vi "Pathfinder.vi"() -> ()   [LabVIEW 2020, in "Data.PG.lvclass"]
uses:
  Data.PG.lvclass
panel:
  out "path_to_selected_column":string="llab_038:d001(TEST_TABLE--new_stuff(hippos))"
  out "table selected":string="TEST_TABLE"
  in  "columns_list":i32(listbox)=1
  in  "Get path":bool
  in  "tables_list":i32(listbox)=34
  in  "STOP":bool
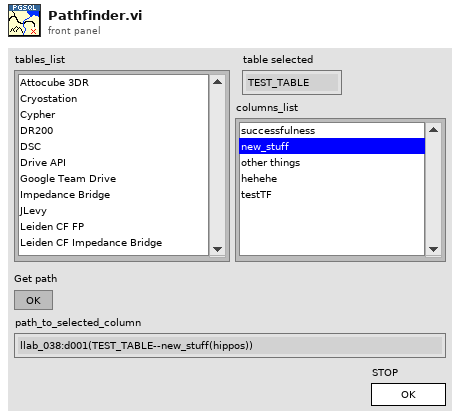
[diagram p1: front panel]
types:
  T1 = enum32{"Invalid", "Standard", "Closed", "Hidden", "Minimized", "Maximized"}
  T2 = enum32{"invalid app kind", "Development System", "Run Time System", "Student Edition", "Embedded LabVIEW", "Evaluation", "Custom"}
  T3 = cluster{"Core":cluster{"Current VI Reference":refnum<vi>, "Close Panel on Exit?":bool}, "Data.PG in":refnum<class "Data.PG.lvclass">, "connection info":cluster{"host":string, "port":string, "dbname":string, "user":string, "password":string}, "table names":string[], "table paths":string[], "column names":string[], "column units":string[], "column paths":string[], "new table name":string, "new column name":string, "new column data type":string, "new column units":string, "selected table":string, "selected column":string, "selected table path":string, "selected column path":string, "Start":timestamp, "End":timestamp, "max points":i32, "selected column units":string}
  T4 = cluster{"host":string, "port":string, "dbname":string, "user":string, "password":string}
  T5 = cluster{"Current VI Reference":refnum<vi>, "Close Panel on Exit?":bool}
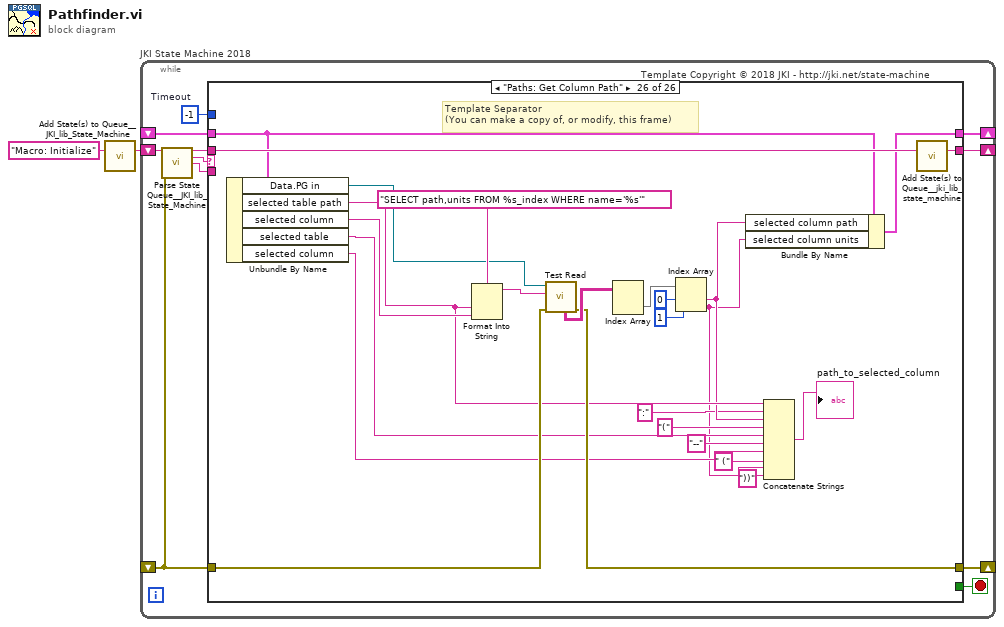
[diagram p0: block diagram]
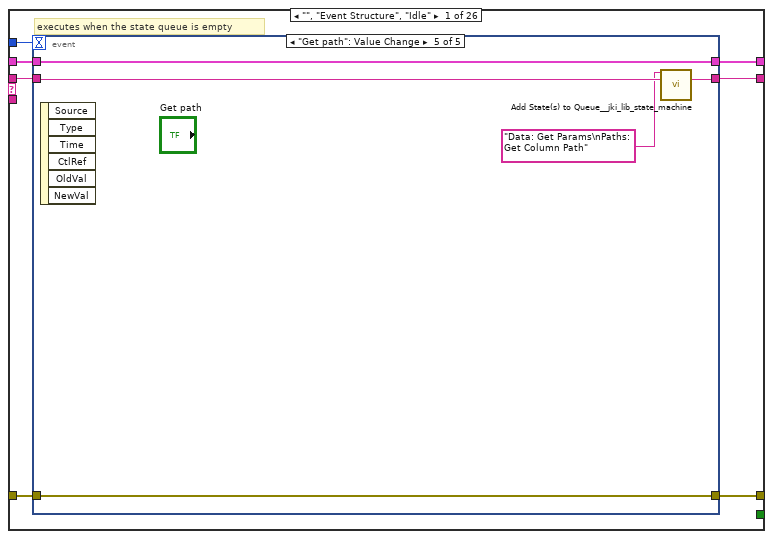
[diagram p2: hidden frame]
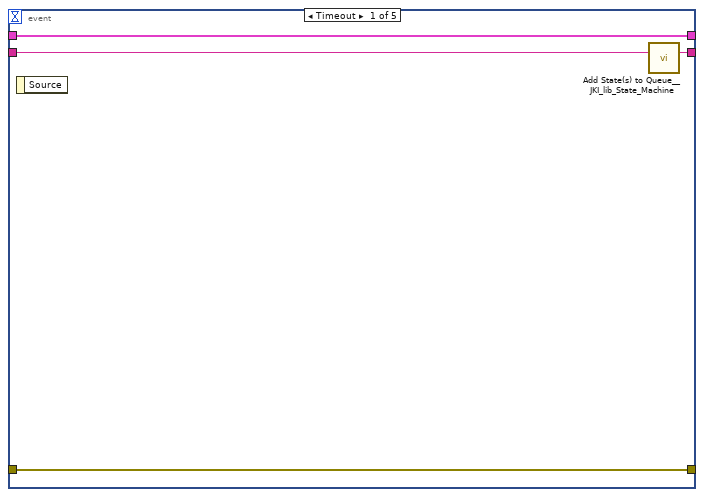
[diagram p3: hidden frame]
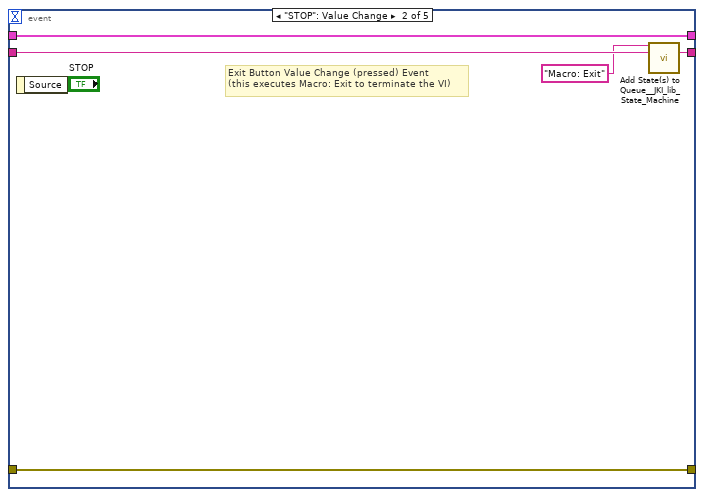
[diagram p4: hidden frame]
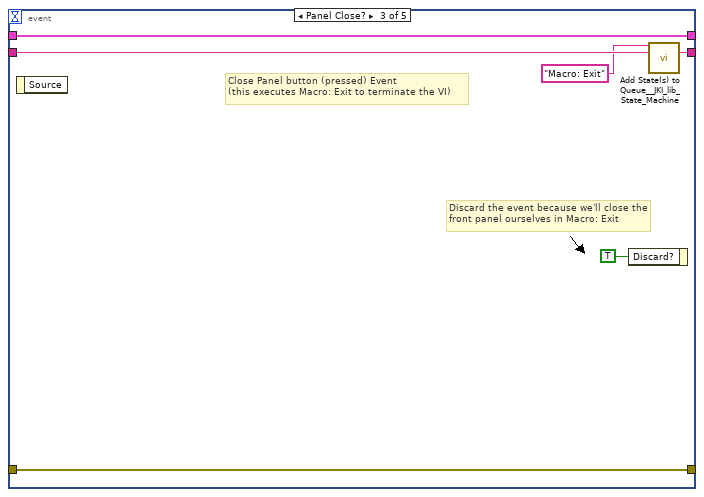
[diagram p5: hidden frame]
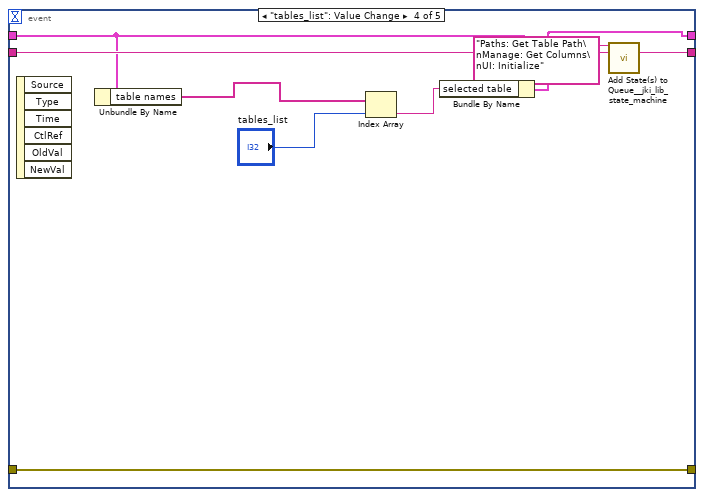
[diagram p6: hidden frame]
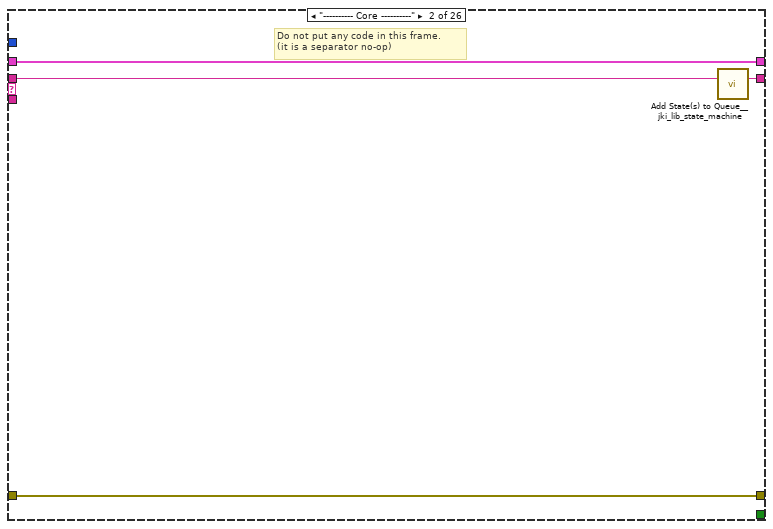
[diagram p7: hidden frame]
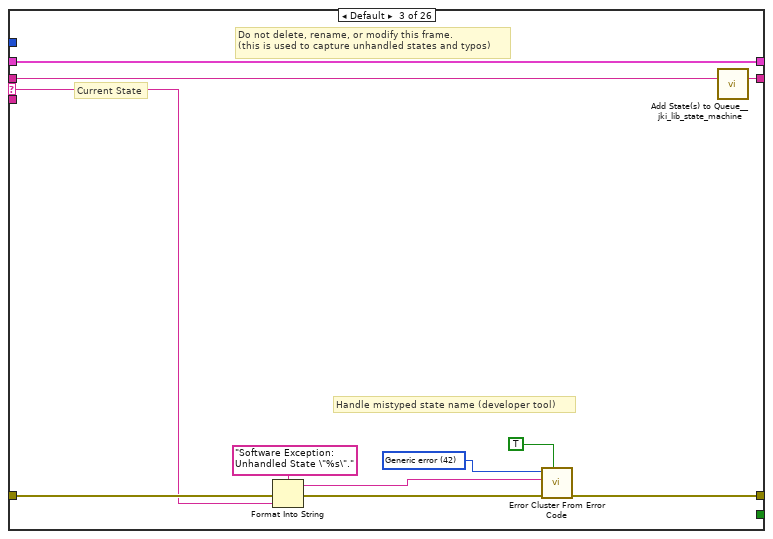
[diagram p8: hidden frame]
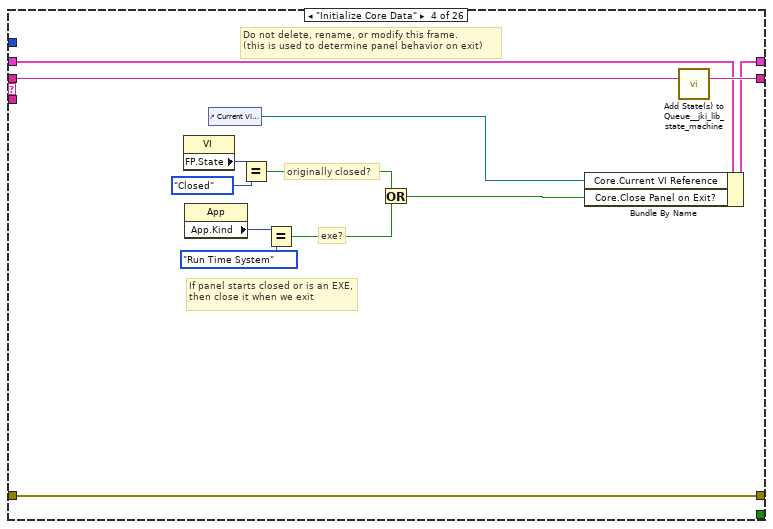
[diagram p9: hidden frame]
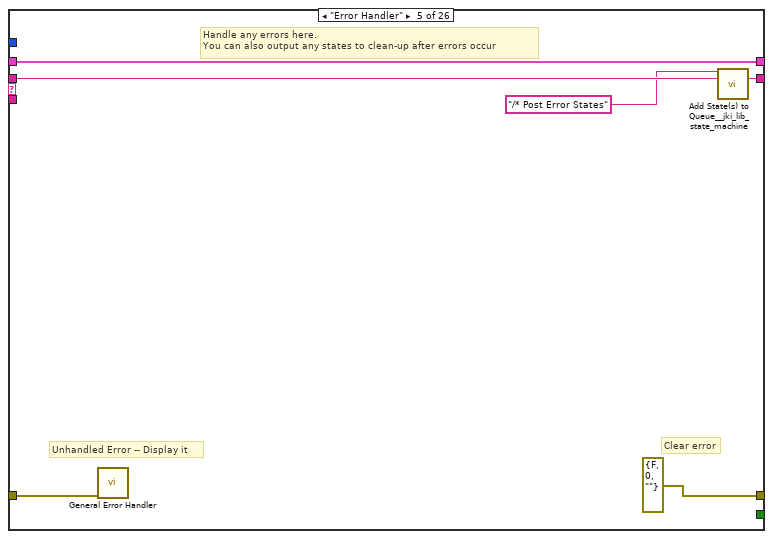
[diagram p10: hidden frame]
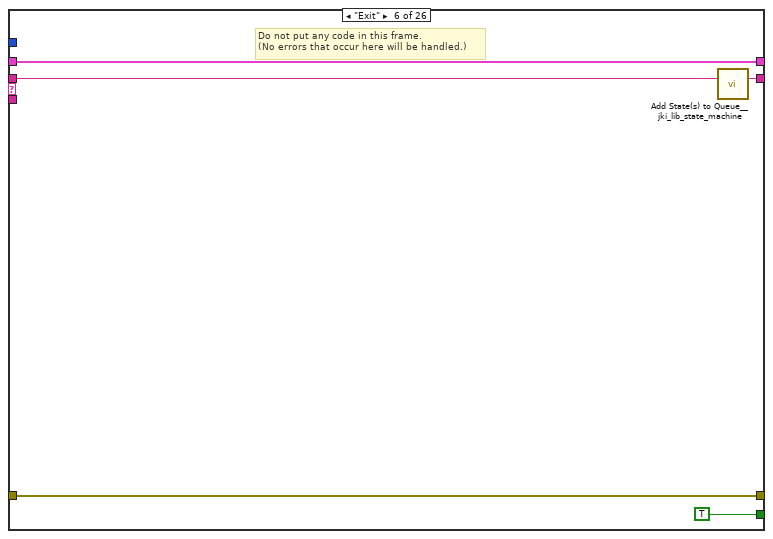
[diagram p11: hidden frame]
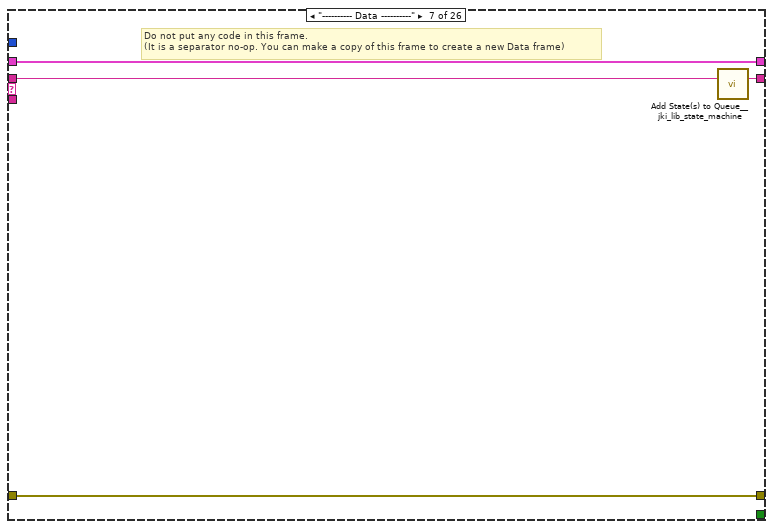
[diagram p12: hidden frame]
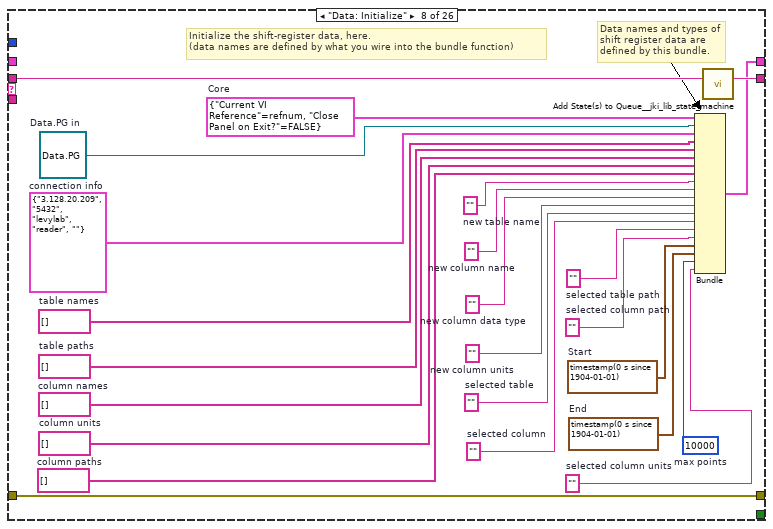
[diagram p13: hidden frame]
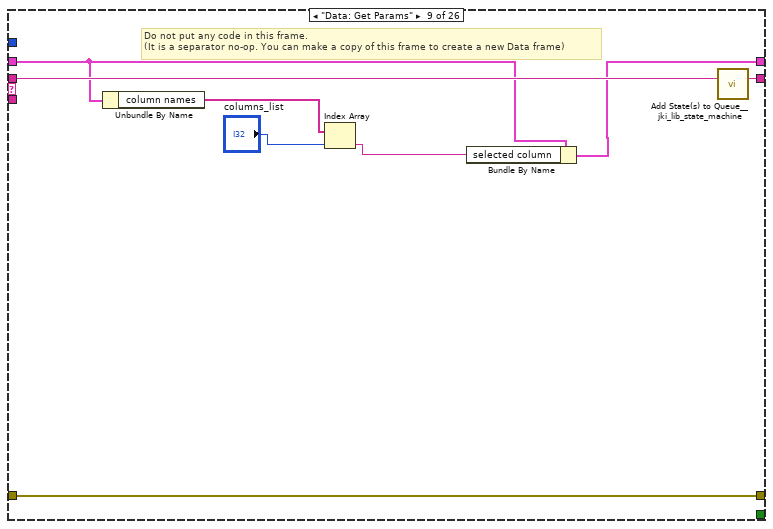
[diagram p14: hidden frame]
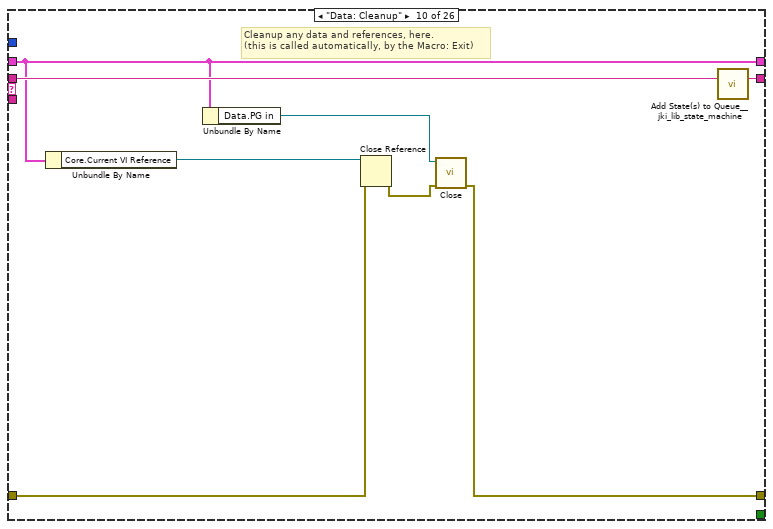
[diagram p15: hidden frame]
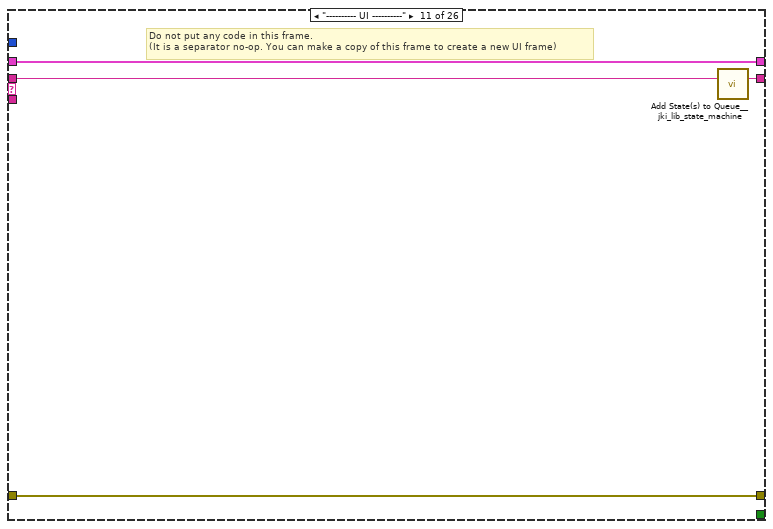
[diagram p16: hidden frame]
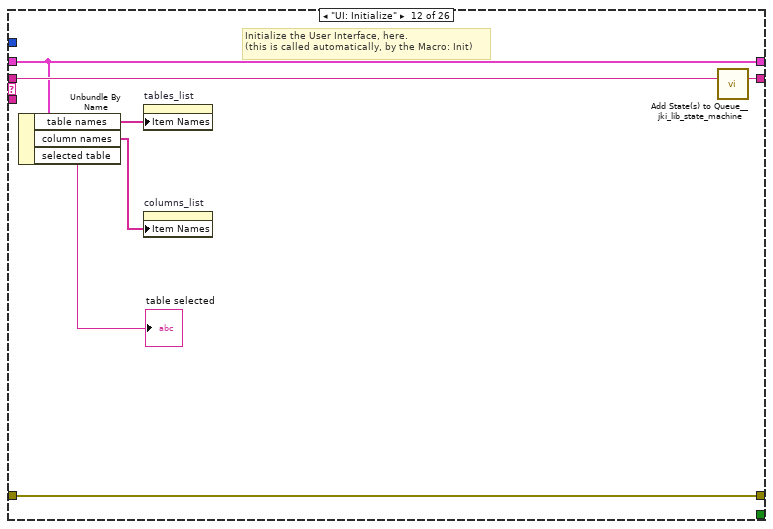
[diagram p17: hidden frame]
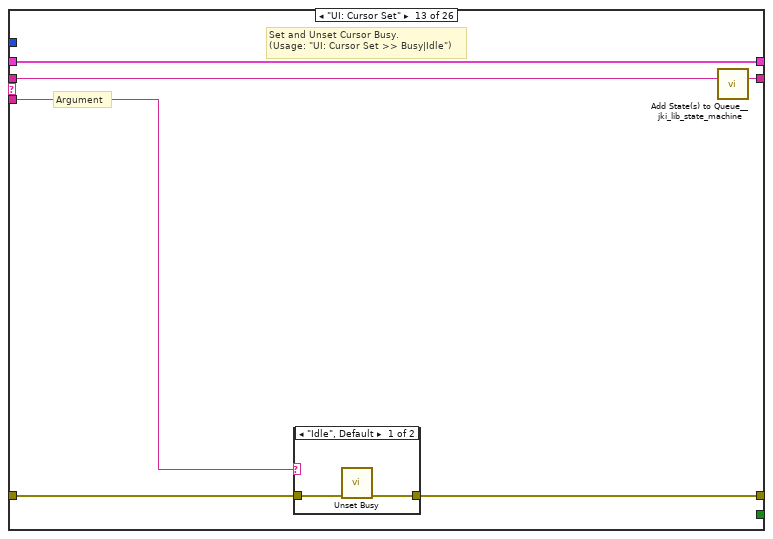
[diagram p18: hidden frame]
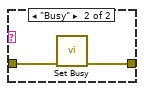
[diagram p19: hidden frame]
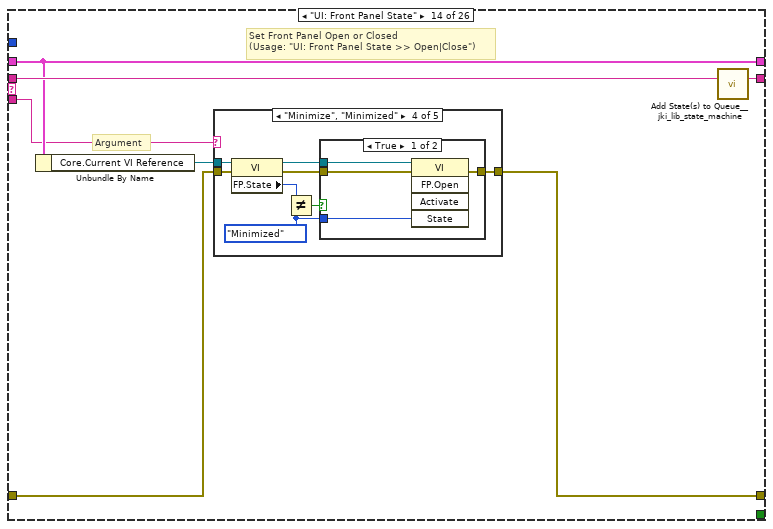
[diagram p20: hidden frame]
diagram:
  n1 = call <vilib>:"Add State(s) to Queue__JKI_lib_State_Machine.vi"("State(s) in (\"\")"="Macro: Initialize") -> ("States Out"=w2:string)  [unwired: 14 in]
  n2 = while "JKI State Machine 2018" {
    shift-right: [w6] -> _
    shift-left: _ -> [w5]
    shift-right: [w9] -> _
    shift-left: _ -> [w3]
    shift-right: [w8] -> _
    shift-left: w2 -> [w10]
    stop <- w7 stop-if-true
    w4 = -1  # Timeout
    # "Template Copyright © 2018 JKI - http://jki.net/state-machine"
    n3 = call <vilib>:"Parse State Queue__JKI_lib_State_Machine.vi"("State Queue"=w10, "Error In (no error)"=w3) -> ("Remaining States"=w12:string, "Current State"=w13:string, "Arguments"=w11:string)  [unwired: 11 in]
    n4 = case shown="\"Paths: Get Column Path\"" w13 {
      selector: w13 -> [_ _ w54 _ _ _ _ _ _ _ _ _ _ _ _ _ _ _ _ _ _ _ _ _ _ _]
      tunnel: w12 -> [w20 w53 w58 w77 w83 w88 w92 w116 w124 w132 w136 w143 w149 w160 w229 w234 w244 w248 w261 w280 w284 w290 w299 w303 w316 w341]
      tunnel: w11 -> [_ _ _ _ _ _ _ _ _ _ _ _ w144 w154 _ _ _ _ _ _ _ _ _ _ _ _]
      tunnel: w5 -> [w18 w50 w56 w70 w80 w86 w89 _ w120 w126 w133 w138 w147 w156 w226 w231 w241 w245 w253 w269 w281 w288 w293 w300 w308 w334]
      tunnel: [w17 w51 w60 w74 errorcluster {"status"=FALSE, "code"=0, "source"=""} ("error out") w85 w90 w113 w122 w127 w134 w141 w145 w157 w227 w232 w242 w246 w255 w263 w282 w285 w294 w301 w304 w331] -> w9
      tunnel: w3 -> [w16 w51 w59 w74 w79 w85 w90 w113 w122 w129 w134 w141 w146 w158 w227 w232 w242 w246 w256 w264 w282 w286 w295 w301 w305 w332]
      tunnel: [w19 w52 w57 w76 w82 w87 w91 w115 w123 w131 w135 w142 w148 w159 w228 w233 w243 w247 w260 w279 w283 w289 w298 w302 w315 w340] -> w8
      tunnel: [_ _ _ _ _ TRUE _ _ _ _ _ _ _ _ _ _ _ _ _ _ _ _ _ _ _ _] -> w7
      tunnel: [w15 w50 w56 w75 w80 w86 w89 w114 w121 w126 w133 w138 w147 w156 w226 w231 w241 w245 w252 w268 w281 w288 w292 w300 w307 w333] -> w6
      tunnel: w4 -> [w14 _ _ _ _ _ _ _ _ _ _ _ _ _ _ _ _ _ _ _ _ _ _ _ _ _]
      frame "", "Event Structure", "Idle" {
        # "executes when the state queue is empty"
        n5 = event shown="[4] \"Get path\": Value Change" {
          selector: _ -> [_ _ _ _ _]
          dyn-events: _ -> [_ _ _ _ _]
          timeout: w14 -> [_ _ _ _ _]
          tunnel: w20 -> [w24 w29 w35 w42 w47]
          tunnel: [w23 w28 w34 w43 w48] -> w19
          tunnel: w18 -> [w21 w26 w32 w38 w49]
          tunnel: [w22 w27 w33 w44 w45] -> w17
          tunnel: w16 -> [w22 w27 w33 w44 w45]
          tunnel: [w21 w26 w32 w37 w49] -> w15
          event Timeout {
            n6 = event-data() -> ()  [unwired: 1 in, 1 out]
            n7 = call <vilib>:"Add State(s) to Queue__JKI_lib_State_Machine.vi"("State(s) in (\"\")"=w24) -> ("States Out"=w23:string)  [unwired: 14 in]
          }
          event "STOP": Value Change {
            # "Exit Button Value Change (pressed) Event\n(this executes Macro: Exit to terminate the VI)"
            n8 = event-data() -> ()  [unwired: 1 in, 1 out]
            n9 = call <vilib>:"Add State(s) to Queue__JKI_lib_State_Machine.vi"("State(s) in Front (\"\")"="Macro: Exit", "State(s) in (\"\")"=w29) -> ("States Out"=w28:string)  [unwired: 13 in]
          }
          event Panel Close? {
            # "Discard the event because we'll close the front panel ourselves in Macro: Exit"
            # "Close Panel button (pressed) Event\n(this executes Macro: Exit to terminate the VI)"
            n10 = event-data() -> ()  [unwired: 1 in, 1 out]
            n11 = event-data("Discard?"=TRUE) -> ()  [unwired: 1 in, 1 out]
            n12 = call <vilib>:"Add State(s) to Queue__JKI_lib_State_Machine.vi"("State(s) in Front (\"\")"="Macro: Exit", "State(s) in (\"\")"=w35) -> ("States Out"=w34:string)  [unwired: 13 in]
          }
          event "tables_list": Value Change {
            n13 = event-data() -> ()  [unwired: 1 in, 6 out]
            n14 = Unbundle By Name(w38) -> ("table names"=w39:string[])
            n15 = Index Array(array=w39, index="tables_list") -> (element=w36:string)
            n16 = Bundle By Name(cluster=w38, "selected table"=w36) -> (w37:T3)
            n17 = call <vilib>:"Add State(s) to Queue__jki_lib_state_machine.vi"("State(s) in Front (\"\")"="Paths: Get Table Path\nManage: Get Columns\nUI: Initialize" ("State(s) in Front (\"\")"), "State(s) in (\"\")"=w42) -> ("States Out"=w43:string)  [unwired: 13 in]
          }
          event "Get path": Value Change {
            n18 = event-data() -> ()  [unwired: 1 in, 6 out]
            n19 = call <vilib>:"Add State(s) to Queue__jki_lib_state_machine.vi"("State(s) in Front (\"\")"="Data: Get Params\nPaths: Get Column Path", "State(s) in (\"\")"=w47) -> ("States Out"=w48:string)  [unwired: 13 in]
          }
        }
      }
      frame "---------- Core ----------" {
        # "Do not put any code in this frame.\n(it is a separator no-op)"
        n20 = call <vilib>:"Add State(s) to Queue__jki_lib_state_machine.vi"("State(s) in (\"\")"=w53) -> ("States Out"=w52:string)  [unwired: 14 in]
      }
      frame Default {
        w63 = 42 items=["No error", "Argument error", "Memory is full", "Out of zone", "End of file", "File already open", "Generic file I/O error", "File not found", "File permission error", "Disk is full", "Duplicate path", "Too many files open", "System feature not enabled", "Resource file not found", "Cannot add resource", "Resource not found", "Image not found", "Image memory error", "Pen does not exist", "Config type invalid", "Config token not found", "Config parse error", "Config memory error", "Bad external code format", "Bad external code offset", "External code not present", "Null window", "Destroy window error", "Null menu", "Print aborted", "Bad print record", "Print driver error", "Windows error during printing", "Memory error during printing", "Print dialog error", "Generic print error", "Invalid device refnum", "Device not found", "Device parameter error", "Device unit error", "Cannot open device", "Device call aborted", "Generic error", "Cancelled by user", "Object ID too low", "Object ID too high", "Object not in heap", "Unknown heap", "Unknown object (invalid DefProc)", "Unknown object (DefProc not in table)", "Message out of range", "Invalid (null) method", "Unknown message", "Manager call not supported", "Bad address", "Network operation in progress", "Network operation timed out", "Connection is busy", "Network attribute not supported", "Network error", "Address in use", "System out of memory", "Connection aborted", "Connection refused", "Not connected", "Already connected", "Connection closed", "Initialization error (interapplication manager)", "Bad occurrence", "Wait on unbound occurrence handler", "Occurrence queue overflow", "Datalog type conflict", "Unused", "Unrecognized type (interapplication manager)", "Memory corrupt", "Failed to make temporary DLL", "Old CIN version", "Drag socket not found", "Failed to load drop-object", "Failed to register OLE object", "Failed to release OLE object", "Format specifier type mismatch", "Unknown format specifier", "Too few format specifiers", "Too many format specifiers", "Scan failed", "Newer CIN version", "Error converting to variant", "Runtime menu error", "Password tampered", "Variant attribute not found", "Incompatible variant data type", "Event data is not available", "Event Store is not present", "Occurrence is not found", "Event Queue is not created", "Event info is not available", "Refnum passed is NULL", "Error retrieving Class GUID", "Error retrieving CoClass GUID", "Error retrieving TypeLib GUID.", "Bad built application magic bytes.", "Specific driver is different from the specific driver associated with the Logical Name.", "There is no session opened to the class driver.", "Max Error", "MAX - Error with config objects", "MAX - Error loading configuration", "MAX - Group not supported"]
        # "Current State"
        # "Do not delete, rename, or modify this frame.\n(this is used to capture unhandled states and typos)"
        # "Handle mistyped state name (developer tool)"
        n21 = Format Into String(format string="Software Exception: Unhandled State \"%s\"." ("message"), error in=w59, w54) -> (resulting string=w62:string, error out=w61:errorcluster)  [unwired: 1 in]
        n22 = call <vilib>:"Error Cluster From Error Code.vi"("show call chain? (False)"=TRUE, "error in (no error)"=w61, "error message (\"\")"=w62, "error code (0)"=w63) -> ("error out"=w60:errorcluster)  [unwired: 5 in]
        n23 = call <vilib>:"Add State(s) to Queue__jki_lib_state_machine.vi"("State(s) in (\"\")"=w58) -> ("States Out"=w57:string)  [unwired: 14 in]
      }
      frame "Initialize Core Data" {
        # "Do not delete, rename, or modify this frame.\n(this is used to determine panel behavior on exit)"
        # "originally closed?"
        # "exe?"
        # "If panel starts closed or is an EXE, then close it when we exit"
        n24 = property class="VI"() -> ("FP.State"=w67:T1)  [unwired: 2 in, 2 out]
        n25 = property class="App"() -> ("App.Kind"=w73:T2)  [unwired: 2 in, 2 out]
        n26 = control-ref of="Current VI Reference"() -> (w68:refnum<vi>)
        n27 = Equal?(x=w67, y=T1."Closed" ("Front Panel Window:State")) -> (x = y?=w65:bool)
        n28 = Equal?(x=w73, y=T2."Run Time System" ("Application:Kind")) -> (x = y?=w71:bool)
        n29 = Or(x=w65, y=w71) -> (x .or. y?=w69:bool)
        n30 = Bundle By Name(cluster=w70, "Core.Current VI Reference"=w68, "Core.Close Panel on Exit?"=w69) -> (w75:T3)
        n31 = call <vilib>:"Add State(s) to Queue__jki_lib_state_machine.vi"("State(s) in (\"\")"=w77) -> ("States Out"=w76:string)  [unwired: 14 in]
      }
      frame "Error Handler" {
        # "Unhandled Error -- Display it"
        # "Handle any errors here.\nYou can also output any states to clean-up after errors occur"
        # "Clear error"
        n32 = call <vilib>:"General Error Handler.vi"("error in (no error)"=w79) -> ()  [unwired: 10 in, 5 out]
        n33 = call <vilib>:"Add State(s) to Queue__jki_lib_state_machine.vi"("State(s) in Front (\"\")"="/* Post Error States", "State(s) in (\"\")"=w83) -> ("States Out"=w82:string)  [unwired: 13 in]
      }
      frame "Exit" {
        # "Do not put any code in this frame.\n(No errors that occur here will be handled.)"
        n34 = call <vilib>:"Add State(s) to Queue__jki_lib_state_machine.vi"("State(s) in (\"\")"=w88) -> ("States Out"=w87:string)  [unwired: 14 in]
      }
      frame "---------- Data ----------" {
        # "Do not put any code in this frame.\n(It is a separator no-op. You can make a copy of this frame to create a new Data frame)"
        n35 = call <vilib>:"Add State(s) to Queue__jki_lib_state_machine.vi"("State(s) in (\"\")"=w92) -> ("States Out"=w91:string)  [unwired: 14 in]
      }
      frame "Data: Initialize" {
        w93 = ""  # selected column units
        w94 = 10000  # max points
        w95 = timestamp(0 s since 1904-01-01)  # End
        w96 = timestamp(0 s since 1904-01-01)  # Start
        w97 = ""  # selected column path
        w98 = ""  # selected table path
        w99 = ""  # selected column
        w100 = ""  # selected table
        w101 = ""  # new column units
        w102 = ""  # new column data type
        w103 = ""  # new column name
        w104 = ""  # new table name
        w105 = string[] []  # column paths
        w106 = string[] []  # column units
        w107 = string[] []  # column names
        w108 = string[] []  # table paths
        w109 = string[] []  # table names
        w110 = T4 {"host"="3.128.20.209", "port"="5432", "dbname"="levylab", "user"="reader", "password"=""}  # connection info
        w111 = refnum<class "Data.PG.lvclass"> refnum  # Data.PG in
        w112 = T5 {"Current VI Reference"=refnum, "Close Panel on Exit?"=FALSE}  # Core
        # "Data names and types of shift register data are defined by this bundle."
        # "Initialize the shift-register data, here.\n(data names are defined by what you wire into the bundle function)"
        n36 = Bundle("Core"=w112, "Data.PG in"=w111, "connection info"=w110, "table names"=w109, "table paths"=w108, "column names"=w107, "column units"=w106, "column paths"=w105, "new table name"=w104, "new column name"=w103, "new column data type"=w102, "new column units"=w101, "selected table"=w100, "selected column"=w99, "selected table path"=w98, "selected column path"=w97, "Start"=w96, "End"=w95, "max points"=w94, "selected column units"=w93) -> (w114:T3)  [unwired: 1 in]
        n37 = call <vilib>:"Add State(s) to Queue__jki_lib_state_machine.vi"("State(s) in (\"\")"=w116) -> ("States Out"=w115:string)  [unwired: 14 in]
      }
      frame "Data: Get Params" {
        # "Do not put any code in this frame.\n(It is a separator no-op. You can make a copy of this frame to create a new Data frame)"
        n38 = Unbundle By Name(w120) -> ("column names"=w118:string[])
        n39 = Index Array(array=w118, index="columns_list") -> (element=w117:string)
        n40 = Bundle By Name(cluster=w120, "selected column"=w117) -> (w121:T3)
        n41 = call <vilib>:"Add State(s) to Queue__jki_lib_state_machine.vi"("State(s) in (\"\")"=w124) -> ("States Out"=w123:string)  [unwired: 14 in]
      }
      frame "Data: Cleanup" {
        # "Cleanup any data and references, here.\n(this is called automatically, by the Macro: Exit)"
        n42 = Unbundle By Name(w126) -> ("Core.Current VI Reference"=w130:refnum<vi>)
        n43 = Unbundle By Name(w126) -> ("Data.PG in"=w125:refnum<class "Data.PG.lvclass">)
        n44 = Close Reference(reference=w130, error in (no error)=w129) -> (error out=w128:errorcluster)
        n45 = call-dynamic "Close.vi"("error in (no error)"=w128, "Data.PG in"=w125) -> ("error out"=w127:errorcluster)  [unwired: 8 in, 1 out]
        n46 = call <vilib>:"Add State(s) to Queue__jki_lib_state_machine.vi"("State(s) in (\"\")"=w132) -> ("States Out"=w131:string)  [unwired: 14 in]
      }
      frame "---------- UI ----------" {
        # "Do not put any code in this frame.\n(It is a separator no-op. You can make a copy of this frame to create a new UI frame)"
        n47 = call <vilib>:"Add State(s) to Queue__jki_lib_state_machine.vi"("State(s) in (\"\")"=w136) -> ("States Out"=w135:string)  [unwired: 14 in]
      }
      frame "UI: Initialize" {
        # "Initialize the User Interface, here.\n(this is called automatically, by the Macro: Init)"
        n48 = Unbundle By Name(w138) -> ("table names"=w140:string[], "column names"=w139:string[], "selected table"=→"table selected":string)
        n49 = property on="tables_list" class="LstBox (strict)"("Item Names"=w140) -> ()  [unwired: 2 in, 2 out]
        n50 = property on="columns_list" class="LstBox (strict)"("Item Names"=w139) -> ()  [unwired: 2 in, 2 out]
        n51 = call <vilib>:"Add State(s) to Queue__jki_lib_state_machine.vi"("State(s) in (\"\")"=w143) -> ("States Out"=w142:string)  [unwired: 14 in]
      }
      frame "UI: Cursor Set" {
        # "Argument"
        # "Set and Unset Cursor Busy.\n(Usage: \"UI: Cursor Set >> Busy|Idle\")"
        n52 = case shown="\"Idle\", Default" w144 {
          tunnel: w146 -> [w151 w153]
          tunnel: [w150 w152] -> w145
          frame "Idle", Default {
            n53 = call <vilib>:"Unset Busy.vi"("error in (no error)"=w151) -> ("error out"=w150:errorcluster)  [unwired: 10 in]
          }
          frame "Busy" {
            n54 = call <vilib>:"Set Busy.vi"("error in (no error)"=w153) -> ("error out"=w152:errorcluster)  [unwired: 9 in, 1 out]
          }
        }
        n55 = call <vilib>:"Add State(s) to Queue__jki_lib_state_machine.vi"("State(s) in (\"\")"=w149) -> ("States Out"=w148:string)  [unwired: 14 in]
      }
      frame "UI: Front Panel State" {
        # "Argument"
        # "Set Front Panel Open or Closed\n(Usage: \"UI: Front Panel State >> Open|Close\")"
        n56 = Unbundle By Name(w156) -> ("Core.Current VI Reference"=w155:refnum<vi>)
        n57 = case shown="\"Minimize\", \"Minimized\"" w154 {
          tunnel: w158 -> [w166 w181 w192 w205 w218]
          tunnel: [w168 w182 w194 w207 w220] -> w157
          tunnel: w155 -> [w167 w179 w193 w206 w219]
          frame "Open", "Standard", Default {
            w161 = T1."Standard" ("State")
            n58 = property class="VI"(reference=w167, error in=w166) -> (reference out=w164:refnum<vi>, error out=w165:errorcluster, "FP.State"=w163:T1)
            n59 = Not Equal?(x=w163, y=w161) -> (x != y?=w162:bool)
            n60 = case shown="True" w162 {
              tunnel: [w172 w174] -> w168
              tunnel: w165 -> [w171 w174]
              tunnel: w164 -> [w170 _]
              tunnel: w161 -> [w169 _]
              frame True {
                n61 = invoke class="VI" method="FP.Open"(reference=w170, error in=w171, "Activate"=TRUE, "State"=w169) -> (error out=w172:errorcluster)  [unwired: 1 in, 4 out]
              }
              frame False {
              }
            }
          }
          frame "Close", "Closed" {
            n62 = property class="VI"(reference=w179, error in=w181) -> (reference out=w178:refnum<vi>, error out=w180:errorcluster, "FP.State"=w176:T1)
            n63 = Not Equal?(x=w176, y=T1."Closed" ("Front Panel Window:State")) -> (x != y?=w175:bool)
            n64 = case shown="True" w175 {
              tunnel: [w183 w186] -> w182
              tunnel: w180 -> [w183 w185]
              tunnel: w178 -> [_ w184]
              frame False {
              }
              frame True {
                n65 = invoke class="VI" method="FP.Close"(reference=w184, error in=w185) -> (error out=w186:errorcluster)  [unwired: 1 in, 2 out]
              }
            }
          }
          frame "Hidden", "Hide" {
            w187 = T1."Hidden" ("State")
            n66 = property class="VI"(reference=w193, error in=w192) -> (reference out=w190:refnum<vi>, error out=w191:errorcluster, "FP.State"=w189:T1)
            n67 = Not Equal?(x=w189, y=w187) -> (x != y?=w188:bool)
            n68 = case shown="True" w188 {
              tunnel: [w198 w199] -> w194
              tunnel: w191 -> [w197 w199]
              tunnel: w190 -> [w196 _]
              tunnel: w187 -> [w195 _]
              frame True {
                n69 = invoke class="VI" method="FP.Open"(reference=w196, error in=w197, "State"=w195) -> (error out=w198:errorcluster)  [unwired: 2 in, 4 out]
              }
              frame False {
              }
            }
          }
          frame "Minimize", "Minimized" {
            w200 = T1."Minimized" ("State")
            n70 = property class="VI"(reference=w206, error in=w205) -> (reference out=w203:refnum<vi>, error out=w204:errorcluster, "FP.State"=w202:T1)
            n71 = Not Equal?(x=w202, y=w200) -> (x != y?=w201:bool)
            n72 = case shown="True" w201 {
              tunnel: [w211 w212] -> w207
              tunnel: w204 -> [w210 w212]
              tunnel: w203 -> [w209 _]
              tunnel: w200 -> [w208 _]
              frame True {
                n73 = invoke class="VI" method="FP.Open"(reference=w209, error in=w210, "State"=w208) -> (error out=w211:errorcluster)  [unwired: 2 in, 4 out]
              }
              frame False {
              }
            }
          }
          frame "Maximize", "Maximized" {
            w213 = T1."Maximized" ("State")
            n74 = property class="VI"(reference=w219, error in=w218) -> (reference out=w216:refnum<vi>, error out=w217:errorcluster, "FP.State"=w215:T1)
            n75 = Not Equal?(x=w215, y=w213) -> (x != y?=w214:bool)
            n76 = case shown="True" w214 {
              tunnel: [w224 w225] -> w220
              tunnel: w217 -> [w223 w225]
              tunnel: w216 -> [w222 _]
              tunnel: w213 -> [w221 _]
              frame True {
                n77 = invoke class="VI" method="FP.Open"(reference=w222, error in=w223, "State"=w221) -> (error out=w224:errorcluster)  [unwired: 2 in, 4 out]
              }
              frame False {
              }
            }
          }
        }
        n78 = call <vilib>:"Add State(s) to Queue__jki_lib_state_machine.vi"("State(s) in (\"\")"=w160) -> ("States Out"=w159:string)  [unwired: 14 in]
      }
      frame "---------- Macro ----------" {
        # "Do not put any code in this frame.\n(It is a separator no-op. You can make a copy of this frame to create a new Macro frame)"
        n79 = call <vilib>:"Add State(s) to Queue__jki_lib_state_machine.vi"("State(s) in (\"\")"=w229) -> ("States Out"=w228:string)  [unwired: 14 in]
      }
      frame "Macro: Initialize" {
        w230 = "Data: Initialize\nInitialize Core Data\nConnection: Open\nManage: Get Tables\nUI: Initialize\nUI: Front Panel State >> Open"  # Data: Initialize Initialize Core Data Connection: Open Manage: Get Tables UI: Initialize UI: Front Panel State >> Open
        # "Initialization Macro\n(This is called once, when the VI starts)"
        n80 = call <vilib>:"Add State(s) to Queue__jki_lib_state_machine.vi"("State(s) in Front (\"\")"=w230, "State(s) in (\"\")"=w234) -> ("States Out"=w233:string)  [unwired: 13 in]
      }
      frame "Macro: Exit" {
        # "Exit Macro\n(This is called once, when the VI exits)"
        n81 = Unbundle By Name(w241) -> ("Core.Close Panel on Exit?"=w240:bool)
        n82 = Select(t="UI: Front Panel State >> Close", s=w240, f="") -> (s? t:f=w237:string)
        n83 = call <vilib>:"Add State(s) to Queue__jki_lib_state_machine.vi"("State(s) in (\"\")"=w237, "State(s) at Back (\"\")"="Data: Cleanup\nConnection: Close\nExit") -> ("States Out"=w235:string)  [unwired: 13 in]
        n84 = call <vilib>:"Add State(s) to Queue__jki_lib_state_machine.vi"("State(s) in Front (\"\")"=w235, "State(s) in (\"\")"=w244) -> ("States Out"=w243:string)  [unwired: 13 in]
      }
      frame "---------- Manage ----------" {
        # "Template Separator\n(You can make a copy of, or modify, this frame)"
        n85 = call <vilib>:"Add State(s) to Queue__jki_lib_state_machine.vi"("State(s) in (\"\")"=w248) -> ("States Out"=w247:string)  [unwired: 14 in]
      }
      frame "Manage: Get Tables" {
        # "Your code here.\n(You can make a copy of, or modify, this frame)"
        n86 = Unbundle By Name(w253) -> ("Data.PG in"=w259:refnum<class "Data.PG.lvclass">)
        n87 = call-dynamic "Test Read.vi"("error in (no error)"=w256, "command"="SELECT * FROM table_index ORDER BY name;", "Data.PG in"=w259) -> ("error out"=w255:errorcluster, "Result"=w257:string[][])  [unwired: 3 in, 4 out]
        n88 = Transpose 2D Array(2D array=w257) -> (transposed array=w254:string[][])
        n89 = Index Array(array=w254, index (row) #2=1 ("index (row)")) -> (element #1=w251:string[], element #2=w249:string[])  [unwired: 3 in]
        n90 = Bundle By Name(cluster=w253, "table names"=w251, "table paths"=w249) -> (w252:T3)
        n91 = call <vilib>:"Add State(s) to Queue__jki_lib_state_machine.vi"("State(s) in (\"\")"=w261) -> ("States Out"=w260:string)  [unwired: 14 in]
      }
      frame "Manage: Get Columns" {
        # "Your code here.\n(You can make a copy of, or modify, this frame)"
        n92 = Unbundle By Name(w269) -> ("Data.PG in"=w278:refnum<class "Data.PG.lvclass">, "selected table path"=w276:string)
        n93 = Format Into String(format string="SELECT * FROM %s_index WHERE name <>'time'; ", w276) -> (resulting string=w275:string)  [unwired: 2 in, 1 out]
        n94 = call-dynamic "Test Read.vi"("error in (no error)"=w264, "command"=w275, "Data.PG in"=w278) -> ("error out"=w263:errorcluster, "Result"=w274:string[][])  [unwired: 3 in, 4 out]
        n95 = Transpose 2D Array(2D array=w274) -> (transposed array=w273:string[][])
        n96 = Index Array(array=w273, index (row) #1=0 ("index (row)"), index (row) #2=1 ("index (row)"), index (row) #3=2 ("index (row)")) -> (element #1=w267:string[], element #2=w266:string[], element #3=w265:string[])  [unwired: 3 in]
        n97 = Bundle By Name(cluster=w269, "column names"=w267, "column units"=w266, "column paths"=w265) -> (w268:T3)
        n98 = call <vilib>:"Add State(s) to Queue__jki_lib_state_machine.vi"("State(s) in Front (\"\")"="UI: Initialize" ("State(s) in Front (\"\")"), "State(s) in (\"\")"=w280) -> ("States Out"=w279:string)  [unwired: 13 in]
      }
      frame "---------- Connection ----------" {
        # "Template Separator\n(You can make a copy of, or modify, this frame)"
        n99 = call <vilib>:"Add State(s) to Queue__jki_lib_state_machine.vi"("State(s) in (\"\")"=w284) -> ("States Out"=w283:string)  [unwired: 14 in]
      }
      frame "Connection: Close" {
        # "Template Separator\n(You can make a copy of, or modify, this frame)"
        n100 = Unbundle By Name(w288) -> ("Data.PG in"=w287:refnum<class "Data.PG.lvclass">)
        n101 = call-dynamic "Close.vi"("error in (no error)"=w286, "Data.PG in"=w287) -> ("error out"=w285:errorcluster)  [unwired: 8 in, 1 out]
        n102 = call <vilib>:"Add State(s) to Queue__jki_lib_state_machine.vi"("State(s) in (\"\")"=w290) -> ("States Out"=w289:string)  [unwired: 14 in]
      }
      frame "Connection: Open" {
        # "Template Separator\n(You can make a copy of, or modify, this frame)"
        n103 = Unbundle By Name(w293) -> ("Data.PG in"=w297:refnum<class "Data.PG.lvclass">, "connection info"=w296:T4)
        n104 = call "Set Connection Info.vi"("error in (no error)"=w295, "connection info"=w296, "Data.PG in"=w297) -> ("error out"=w294:errorcluster, "Data.PG out"=w291:refnum<class "Data.PG.lvclass">)  [unwired: 7 in]
        n105 = Bundle By Name(cluster=w293, "Data.PG in"=w291) -> (w292:T3)
        n106 = call <vilib>:"Add State(s) to Queue__jki_lib_state_machine.vi"("State(s) in (\"\")"=w299) -> ("States Out"=w298:string)  [unwired: 14 in]
      }
      frame "---------- Paths ----------" {
        # "Template Separator\n(You can make a copy of, or modify, this frame)"
        n107 = call <vilib>:"Add State(s) to Queue__jki_lib_state_machine.vi"("State(s) in (\"\")"=w303) -> ("States Out"=w302:string)  [unwired: 14 in]
      }
      frame "Paths: Get Table Path" {
        # "Template Separator\n(You can make a copy of, or modify, this frame)"
        n108 = Unbundle By Name(w308) -> ("Data.PG in"=w313:refnum<class "Data.PG.lvclass">, "selected table"=w311:string)
        n109 = Format Into String(format string="SELECT path FROM table_index WHERE name='%s'", w311) -> (resulting string=w312:string)  [unwired: 2 in, 1 out]
        n110 = call-dynamic "Test Read.vi"("error in (no error)"=w305, "command"=w312, "Data.PG in"=w313) -> ("error out"=w304:errorcluster, "Result"=w310:string[][])  [unwired: 3 in, 4 out]
        n111 = Index Array(array=w310) -> (element=w309:string[])  [unwired: 2 in]
        n112 = Index Array(array=w309) -> (element=w306:string)  [unwired: 1 in]
        n113 = Bundle By Name(cluster=w308, "selected table path"=w306) -> (w307:T3)
        n114 = call <vilib>:"Add State(s) to Queue__jki_lib_state_machine.vi"("State(s) in (\"\")"=w316) -> ("States Out"=w315:string)  [unwired: 14 in]
      }
      frame "Paths: Get Column Path" {
        # "Template Separator\n(You can make a copy of, or modify, this frame)"
        n115 = Unbundle By Name(w334) -> ("Data.PG in"=w338:refnum<class "Data.PG.lvclass">, "selected table path"=w327:string, "selected column"=w330:string, "selected table"=w322:string, "selected column"=w320:string)
        n116 = Format Into String(format string="SELECT path,units FROM %s_index WHERE name='%s'", w327, w330) -> (resulting string=w337:string)  [unwired: 2 in, 1 out]
        n117 = call-dynamic "Test Read.vi"("error in (no error)"=w332, "command"=w337, "Data.PG in"=w338) -> ("error out"=w331:errorcluster, "Result"=w336:string[][])  [unwired: 3 in, 4 out]
        n118 = Index Array(array=w336) -> (element=w335:string[])  [unwired: 2 in]
        n119 = Index Array(array=w335, index #1=0 ("index"), index #2=1 ("index")) -> (element #1=w325:string, element #2=w318:string)
        n120 = Bundle By Name(cluster=w334, "selected column path"=w325, "selected column units"=w318) -> (w333:T3)
        n121 = Concatenate Strings(w327, ":" ("string"), w325, "(" ("string"), w322, "--" ("string"), w320, " (" ("string"), w318, "))" ("string")) -> (→"path_to_selected_column":string)
        n122 = call <vilib>:"Add State(s) to Queue__jki_lib_state_machine.vi"("State(s) in (\"\")"=w341) -> ("States Out"=w340:string)  [unwired: 14 in]
      }
    }
  }
